vi "BreadcrumbNavigator Tester.vi"() -> ()   [LabVIEW 2015]
uses:
  <vilib>/QSI/QControls/QControl Classes/BreadcrumbNavigator/BreadcrumbNavigator.lvclass
panel:
  in  "Item Name to Add":string
  out "ClickedItem":string
  in  "Add Item":bool
  out "Breadcrumb Navigation":string
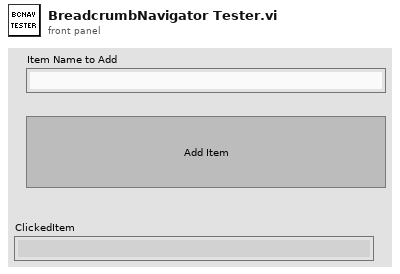
[diagram p1: front panel]
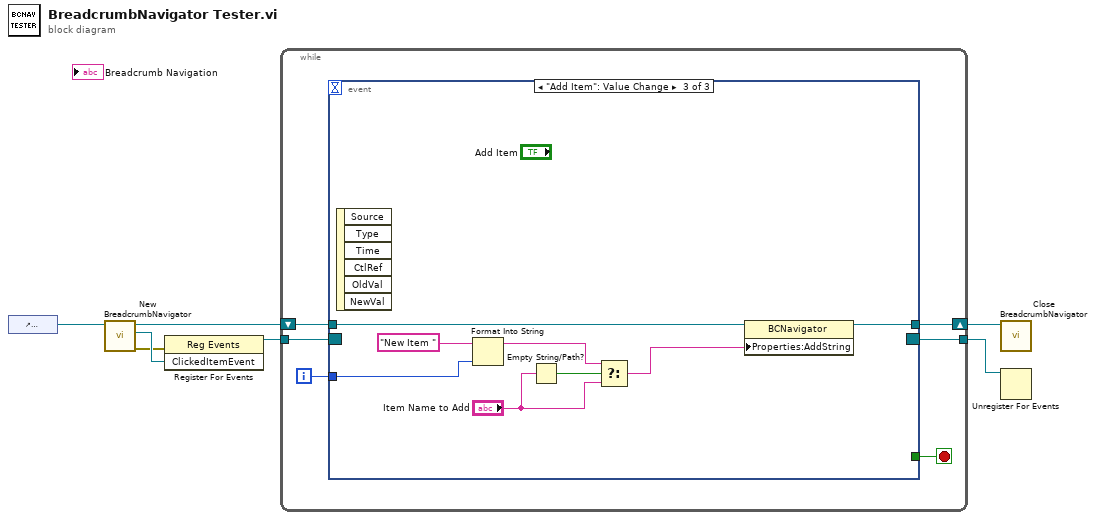
[diagram p0: block diagram]
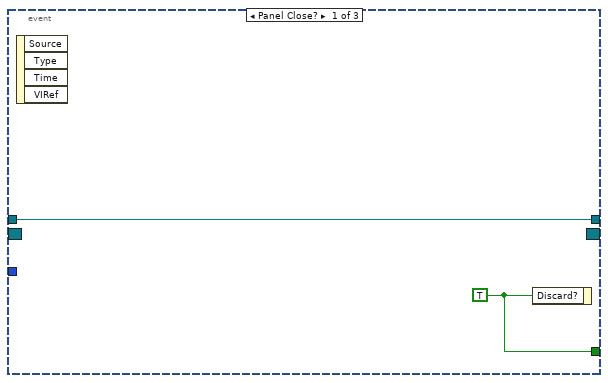
[diagram p2: hidden frame]
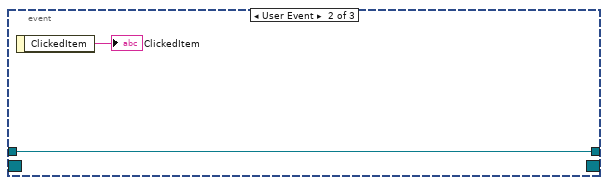
[diagram p3: hidden frame]
diagram:
  n1 = control-ref of="Breadcrumb Navigation"() -> (w7:refnum<vi>)
  n2 = call <vilib>:"New BreadcrumbNavigator.vi"("Reference"=w7) -> ("error out"=w3:errorcluster, "ClickedItemEvent"=w4:refnum<user-event>, "BreadcrumbNavigation out"=w6:refnum<class "BreadcrumbNavigator.lvclass">)  [unwired: 8 in]
  n3 = register-events(error in=w3, w4) -> (reference out=w2:refnum<event-registration>)  [unwired: 1 in, 1 out]
  n4 = while {
    shift-right: [w12] -> w5
    shift-left: w6 -> [w11]
    tunnel: w2 -> [w10]
    tunnel: [w9] -> w1
    i -> [w8]
    stop <- w13 stop-if-true
    n5 = event shown="[2] \"Add Item\": Value Change" {
      selector: w10 -> [_ _ _]
      dyn-events: [_ _ _] -> w9
      timeout: _ -> [_ _ _]
      tunnel: [w15 _ _] -> w13
      tunnel: [w14 w17 w24] -> w12
      tunnel: w11 -> [w14 w17 w25]
      tunnel: w8 -> [_ _ w20]
      event Panel Close? {
        w15 = TRUE ("Discard?")
        n6 = event-data() -> ()  [unwired: 1 in, 4 out]
        n7 = event-data("Discard?"=w15) -> ()  [unwired: 1 in, 1 out]
      }
      event User Event {
        n8 = event-data() -> ("ClickedItem"=→"ClickedItem":string)  [unwired: 1 in]
      }
      event "Add Item": Value Change {
        n9 = event-data() -> ()  [unwired: 1 in, 6 out]
        n10 = Format Into String(initial string="New Item " ("t"), w20) -> (resulting string=w19:string)  [unwired: 2 in, 1 out]
        n11 = Empty String/Path?(string/path="Item Name to Add") -> (empty?=w23:bool)
        n12 = Select(t=w19, s=w23, f="Item Name to Add") -> (s? t:f=w18:string)
        n13 = property class="BCNavigator"(reference=w25, "Properties:AddString"=w18) -> (reference out=w24:refnum<class "BreadcrumbNavigator.lvclass">)  [unwired: 1 in, 1 out]
      }
    }
  }
  n14 = call <vilib>:"Close BreadcrumbNavigator.vi"("BreadcrumbNavigation in"=w5) -> ()  [unwired: 10 in, 1 out]
  n15 = Unregister For Events(event registration refnum=w1) -> ()  [unwired: 1 in, 1 out]
